vi "generateRTPRBS.vi"(0 "Utilities in":refnum<class "Utilities.lvclass">, 1 "W":dbl=2.0, 3 "Th":dbl=0.02 format="%#_13g", 5 "MAX":dbl=3.0 format="%#_13g", 7 "activate":bool, 9 "MIN":dbl=2.0 format="%#_13g", 11 "error in (no error)":errorcluster, 12 "PRBS samples":i32=800) -> (4 "Utilities out":refnum<class "Utilities.lvclass">, 6 "Val":dbl, 8 "Size":i32, 10 "totalSize":i32, 15 "error out":errorcluster)   [LabVIEW 2023, in "Utilities.lvclass"]
uses:
  Utilities.lvclass
  <vilib>/Analysis/1siggen.llb/Ramp Pattern by Samples.vi
  <vilib>/numeric/Random Number (Range) I64.vi
  <vilib>/numeric/sub_Random U32.vi
  <vilib>/Analysis/1siggen.llb/Ramp Pattern by Delta.vi
  <vilib>/Analysis/NI_AALBase.lvlib
  <vilib>/ptbypt/NI_PtbyPt.lvlib
panel:
  in  "Save":bool
  in  "stop":bool
  out "element":dbl
  out "XY Graph":cluster{dbl, dbl}[](graph)
  out "cos(x)":dbl[](array[numeric])
  in  "time":dbl=0.2 format="%#_13g"
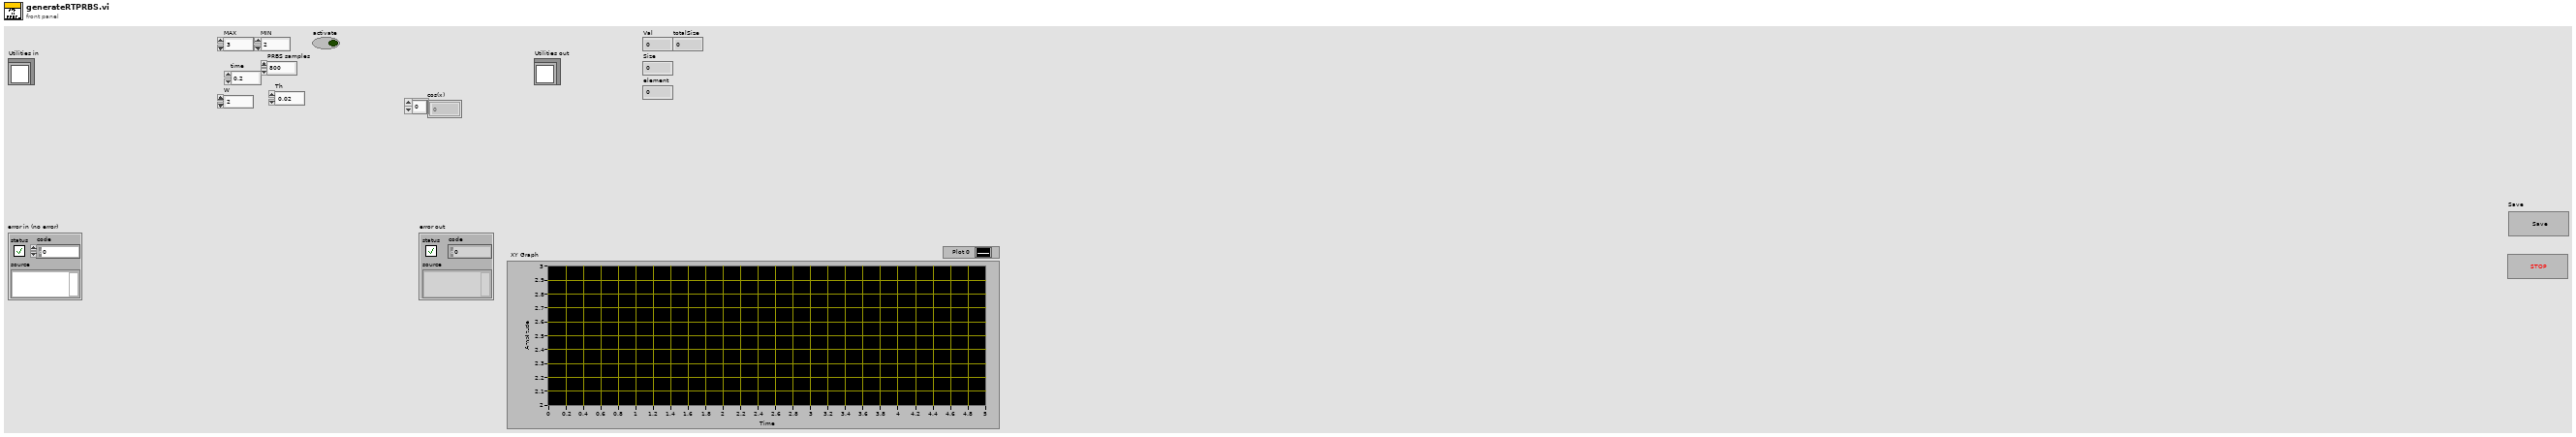
[diagram p1: front panel]
types:
  T1 = typedef "imagedata.ctl" = cluster{"image type":i32, "image depth":i32, "image":u8[], "mask":u8[], "colors":u32[], "Rectangle":cluster{"left":i16, "top":i16, "right":i16, "bottom":i16}}
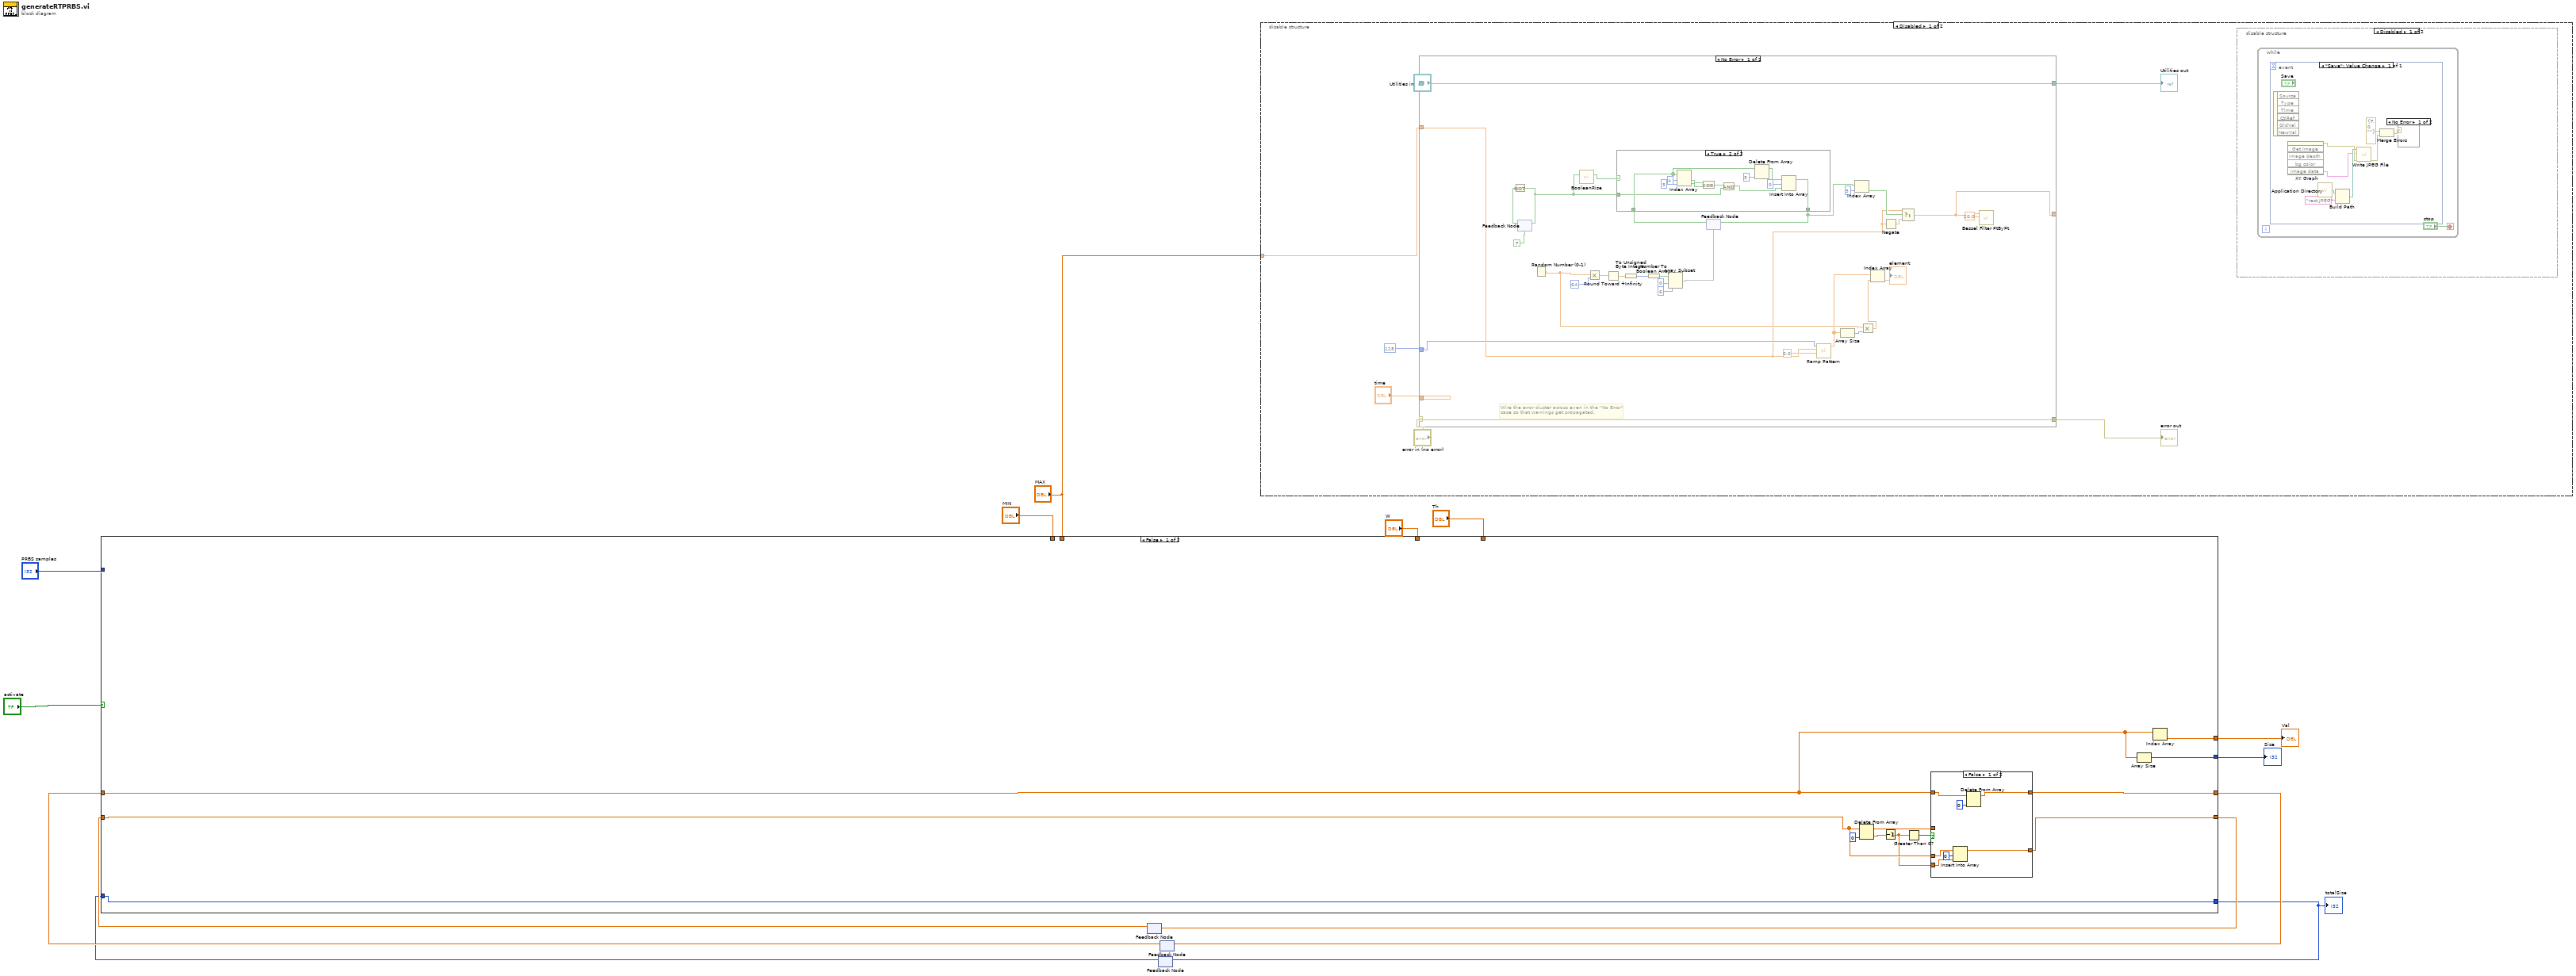
[diagram p0: block diagram]
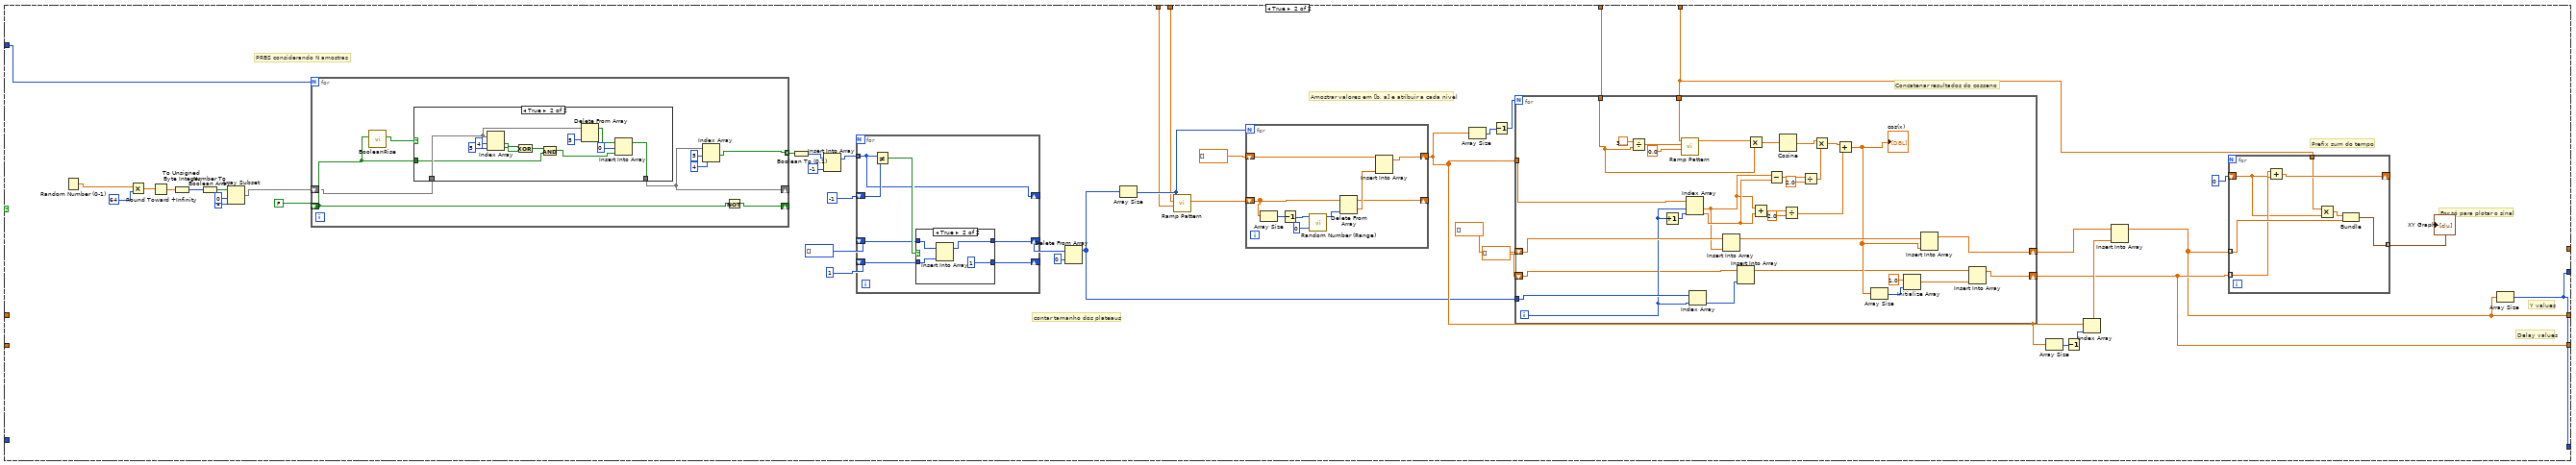
[diagram p8: hidden frame]
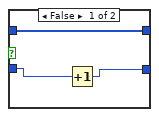
[diagram p10: hidden frame]
diagram:
  n1 = feedback #1() -> (w13:dbl[])  [unwired: 1 in]
  n2 = feedback #2() -> (w1:i32)  [unwired: 1 in]
  n3 = feedback #3() -> (w11:dbl[])  [unwired: 1 in]
  n4 = case shown="False" "activate" {
    tunnel: [w19 w37] -> w12
    tunnel: [w21 w44] -> w14
    tunnel: w13 -> [w23 _]
    tunnel: w11 -> [w17 _]
    tunnel: [w18 _] -> w3
    tunnel: "Th" -> [_ w42]
    tunnel: "W" -> [_ w41]
    tunnel: "MAX" -> [_ w40]
    tunnel: "MIN" -> [_ w39]
    tunnel: "PRBS samples" -> [_ w38]
    tunnel: [w16 w36] -> w5
    tunnel: [w15 w36] -> w2
    tunnel: w1 -> [w15 _]
    frame False {
      n5 = Delete From Array(array=w23, index=0) -> (deleted portion=w26:dbl, array with subset deleted=w24:dbl[])  [unwired: 1 in]
      n6 = Decrement(x=w26) -> (x-1=w22:dbl)
      n7 = Greater Than 0?(x=w22) -> (x > 0?=w25:bool)
      n8 = case shown="False" w25 {
        tunnel: w24 -> [_ w35]
        tunnel: w23 -> [w33 _]
        tunnel: w22 -> [w32 _]
        tunnel: [w31 w35] -> w21
        tunnel: w17 -> [w29 w34]
        tunnel: [w27 w34] -> w19
        frame False {
          n9 = Insert Into Array(array=w33, index=0, new element=w32) -> (w31:dbl[])
          n10 = Delete From Array(array=w29, index=0) -> (array with subset deleted=w27:dbl[])  [unwired: 1 in, 1 out]
        }
        frame True {
        }
      }
      n11 = Array Size(array=w17) -> (size(s)=w16:i32)
      n12 = Index Array(array=w17) -> (element=w18:dbl)  [unwired: 1 in]
    }
    frame True {
      # "For só para plotar o sinal"
      # "Delay values"
      # "Y values"
      # "Prefix sum do tempo"
      # "Concatenar resultados do cosseno"
      # "Amostrar valores em [b, a] e atribuir a cada nivel"
      # "contar tamanho dos plateaus"
      # "PRBS considerando N amostras"
      n13 = Random Number (0-1)() -> (number: 0 to 1=w48:dbl)
      n14 = Multiply(x=w48, y=64) -> (x*y=w71:dbl)
      n15 = Round Toward +Infinity(x=w71) -> (ceil(x): smallest int >= x=w73:dbl)
      n16 = To Unsigned Byte Integer(number=w73) -> (unsigned 8bit integer=w74:u8)
      n17 = Number To Boolean Array(number=w74) -> (Boolean array=w75:bool[])
      n18 = Array Subset(array=w75, index=0, length=6) -> (w49:bool[])
      n19 = for {
        N: w38 -> [_]
        shift-right: [w91] -> _
        shift-left: FALSE -> [w92]
        tunnel: [w89] -> w64 mode=indexing
        shift-right: [w88] -> _
        shift-left: w49 -> [w87]
        n20 = call "BooleanRise.vi"("Boolean in"=w92) -> ("Boolean"=w93:bool)  [unwired: 8 in, 2 out]
        n21 = case shown="True" w93 {
          tunnel: [w95 w106] -> w88
          tunnel: w87 -> [w95 w98]
          tunnel: w92 -> [_ w96]
          frame False {
          }
          frame True {
            n22 = Index Array(array=w98, index #1=4 ("index"), index #2=5 ("index")) -> (element #1=w101:bool, element #2=w102:bool)
            n23 = Exclusive Or(1:w102, 2:w101) -> (0:w97:bool)
            n24 = And(x=w97, y=w96) -> ()  [unwired: 1 out]
            n25 = Delete From Array(array=w98, index=5) -> (array with subset deleted=w104:bool[])  [unwired: 1 in, 1 out]
            n26 = Insert Into Array(array=w104, index=0, new element=w97) -> (w106:bool[])
          }
        }
        n27 = Index Array(array=w88, index #1=5 ("index"), index #2=4 ("index")) -> (element #1=w89:bool)  [unwired: 1 out]
        n28 = Not(x=w92) -> (.not. x?=w91:bool)
      }
      n29 = Boolean To (0,1)(Boolean=w64) -> (0, 1=w63:i16[])
      n30 = Insert Into Array(array=w63, new element=i16 -1 ("new element/subarray")) -> (w61:i16[])  [unwired: 1 in]
      n31 = for {
        shift-right: [w146] -> _
        shift-left: -1 -> [w152]
        shift-right: [w147] -> _
        shift-left: 1 -> [w150]
        shift-right: [w148] -> w66
        shift-left: i32[] [] -> [w149]
        tunnel: w61 -> [w146] mode=indexing
        n32 = Not Equal?(x=w146, y=w152) -> (x != y?=w151:bool)
        n33 = case shown="True" w151 {
          tunnel: w150 -> [w155 w158]
          tunnel: w149 -> [w153 w159]
          tunnel: [w153 w157] -> w148
          tunnel: [w154 1] -> w147
          frame False {
            n34 = Increment(x=w155) -> (x+1=w154:i32)
          }
          frame True {
            n35 = Insert Into Array(array=w159, new element=w158) -> (w157:i32[])  [unwired: 1 in]
          }
        }
      }
      n36 = Delete From Array(array=w66, index=0) -> (array with subset deleted=w46:i32[])  [unwired: 1 in, 1 out]
      n37 = Array Size(array=w46) -> (size(s)=w47:i32)
      n38 = call-poly <vilib>:"Ramp Pattern.vi"("start"=w39, "end"=w40, "samples"=w47) -> ("Ramp Pattern"=w60:dbl[])  [unwired: 7 in, 1 out]
      n39 = for {
        N: w47 -> [_]
        shift-right: [w83] -> _
        shift-left: w60 -> [w80]
        shift-right: [w84] -> w53
        shift-left: dbl[] [] ("Ramp Pattern") -> [w86]
        n40 = Array Size(array=w80) -> (size(s)=w82:i32)
        n41 = Decrement(x=w82) -> (x-1=w81:i32)
        n42 = call-poly <vilib>:"Random Number (Range).vi"("lower bound (-100)"=i64 0, "upper bound (100)"=w81) -> ("number"=w78:i64)  [unwired: 9 in]
        n43 = Delete From Array(array=w80, index=w78) -> (deleted portion=w85:dbl, array with subset deleted=w83:dbl[])  [unwired: 1 in]
        n44 = Insert Into Array(array=w86, new element=w85) -> (w84:dbl[])  [unwired: 1 in]
      }
      n45 = Array Size(array=w53) -> (size(s)=w58:i32)
      n46 = Decrement(x=w58) -> (x-1=w57:i32)
      n47 = for {
        N: w57 -> [_]
        tunnel: w53 -> [w145]
        tunnel: w41 -> [w132]
        tunnel: w42 -> [w129]
        shift-right: [w124] -> w44
        shift-left: dbl[] [] -> [w116]
        shift-right: [w119] -> w55
        shift-left: dbl[] [] ("Ramp Pattern") -> [w123]
        tunnel: w46 -> [w118]
        i -> [w117]
        n48 = Divide(x=3.141592653589793, y=w132) -> (x/y=w135:dbl)
        n49 = Increment(x=w117) -> (x+1=w144:i32)
        n50 = call-poly <vilib>:"Ramp Pattern.vi"("start"=0.0, "end"=w135, "delta"=w129) -> ("Ramp Pattern"=w136:dbl[])  [unwired: 6 in, 2 out]
        n51 = Index Array(array=w145, index #1=w117, index #2=w144) -> (element #1=w122:dbl, element #2=w128:dbl)
        n52 = Index Array(array=w118, index=w117) -> (element=w115:i32)
        n53 = Insert Into Array(array=w123, new element=w122) -> (w121:dbl[])  [unwired: 1 in]
        n54 = Insert Into Array(array=w116, new element=w115) -> (w114:dbl[])  [unwired: 1 in]
        n55 = Multiply(x=w136, y=w132) -> (x*y=w137:dbl[])
        n56 = Add(x=w122, y=w128) -> (x+y=w138:dbl)
        n57 = Subtract(x=w122, y=w128) -> (x-y=w139:dbl)
        n58 = Cosine(x=w137) -> (cos(x)=w140:dbl[])
        n59 = Divide(x=w138, y=2.0) -> (x/y=w143:dbl)
        n60 = Divide(x=w139, y=2.0) -> (x/y=w141:dbl)
        n61 = Multiply(x=w140, y=w141) -> (x*y=w142:dbl[])
        n62 = Add(x=w142, y=w143) -> (x+y=w120:dbl[])
        "cos(x)" <- w120
        n63 = Array Size(array=w120) -> (size(s)=w126:i32)
        n64 = Initialize Array(1.0 ("element"), w126) -> (w125:dbl[])
        n65 = Insert Into Array(array=w121, new element=w120) -> (w119:dbl[])  [unwired: 1 in]
        n66 = Insert Into Array(array=w114, new element=w125) -> (w124:dbl[])  [unwired: 1 in]
      }
      n67 = Array Size(array=w53) -> (size(s)=w52:i32)
      n68 = Decrement(x=w52) -> (x-1=w51:i32)
      n69 = Index Array(array=w53, index=w51) -> (element=w54:dbl)
      n70 = Insert Into Array(array=w55, new element=w54) -> (w37:dbl[])  [unwired: 1 in]
      n71 = for {
        tunnel: w37 -> [w112] mode=indexing
        tunnel: w44 -> [w111] mode=indexing
        tunnel: [w113] -> w43 mode=indexing
        shift-right: [w110] -> _
        shift-left: 0 -> [w109]
        tunnel: w42 -> [w108]
        n72 = Add(x=w109, y=w111) -> (x+y=w110:dbl)
        n73 = Multiply(x=w108, y=w109) -> (x*y=w107:dbl)
        n74 = Bundle(w107, w112) -> (w113:cluster{dbl, dbl})  [unwired: 1 in]
      }
      "XY Graph" <- w43
      n75 = Array Size(array=w37) -> (size(s)=w36:i32)
    }
  }
  "Val" <- w3
  "Size" <- w5
  "totalSize" <- w2
  n76 = feedback-in #1(w14) -> ()
  n77 = feedback-in #2(w2) -> ()
  n78 = feedback-in #3(w12) -> ()
  n79 = disable-structure shown="Disabled" {
    disable-tunnel: "MAX" -> [w160 _]
    frame Disabled {
      n80 = case shown="No Error" "error in (no error)" {
        selector: "error in (no error)" -> [w203 w218]
        tunnel: [w203 w218] -> w165
        tunnel: [w204 w217] -> w163
        tunnel: "Utilities in" -> [w204 w217]
        tunnel: w160 -> [w177 _]
        tunnel: "time" -> [_ _]
        tunnel: 128 -> [w185 _]
        tunnel: [w178 _] -> _
        frame No Error {
          # "Wire the error cluster across even in the \"No Error\"\ncase so that warnings get propagated."
          n81 = feedback #4(FALSE) -> (w191:bool)
          n82 = Not(x=w191) -> (.not. x?=w186:bool)
          n83 = feedback-in #4(w186) -> ()
          n84 = Random Number (0-1)() -> (number: 0 to 1=w181:dbl)
          n85 = call "BooleanRise.vi"("Boolean in"=w186) -> ("Boolean"=w187:bool)  [unwired: 8 in, 2 out]
          n86 = Multiply(x=w181, y=64) -> (x*y=w193:dbl)
          n87 = Round Toward +Infinity(x=w193) -> (ceil(x): smallest int >= x=w195:dbl)
          n88 = To Unsigned Byte Integer(number=w195) -> (unsigned 8bit integer=w196:u8)
          n89 = Number To Boolean Array(number=w196) -> (Boolean array=w197:bool[])
          n90 = Array Subset(array=w197, index=0, length=6) -> (w200:bool[])
          n91 = feedback #5(w200) -> (w201:bool[])
          n92 = case shown="True" w187 {
            tunnel: [w205 w216] -> w190
            tunnel: w201 -> [w205 w208]
            tunnel: w186 -> [_ w206]
            frame False {
            }
            frame True {
              n93 = Index Array(array=w208, index #1=4 ("index"), index #2=5 ("index")) -> (element #1=w211:bool, element #2=w212:bool)
              n94 = Exclusive Or(1:w212, 2:w211) -> (0:w207:bool)
              n95 = And(x=w207, y=w206) -> ()  [unwired: 1 out]
              n96 = Delete From Array(array=w208, index=5) -> (array with subset deleted=w214:bool[])  [unwired: 1 in, 1 out]
              n97 = Insert Into Array(array=w214, index=0, new element=w207) -> (w216:bool[])
            }
          }
          n98 = feedback-in #5(w190) -> ()
          n99 = call-poly <vilib>:"Ramp Pattern.vi"("start"=0.0, "end"=w177, "samples"=w185) -> ("Ramp Pattern"=w183:dbl[])  [unwired: 7 in, 1 out]
          n100 = Array Size(array=w183) -> (size(s)=w182:i32)
          n101 = Index Array(array=w190, index=5) -> (element=w188:bool)
          n102 = Multiply(x=w181, y=w182) -> (x*y=w180:dbl)
          n103 = Index Array(array=w183, index=w180) -> (element=→"element":dbl)
          n104 = Negate(x=w177) -> (-x=w202:dbl)
          n105 = Select(t=w177, s=w188, f=w202) -> (s? t:f=w178:dbl)
          n106 = call <vilib>:"Bessel Filter PtByPt.vi"("sampling freq: fs"=20.0, "x"=w178) -> ()  [unwired: 7 in, 2 out]
        }
        frame Error {
        }
      }
      "error out" <- w165
      "Utilities out" <- w163
      n107 = disable-structure shown="Disabled" {
        frame Disabled {
          n108 = while {
            stop <- "stop" stop-if-true
            n109 = event shown="[0] \"Save\": Value Change" {
              selector: _ -> [_]
              dyn-events: _ -> [_]
              timeout: _ -> [_]
              event "Save": Value Change {
                n110 = event-data() -> ()  [unwired: 1 in, 6 out]
                n111 = invoke on="XY Graph" class="XYGraph (strict)" method="Get Image"() -> (error out=w170:errorcluster, "image data"=w169:T1)  [unwired: 6 in, 4 out]
                n112 = call <vilib>:"Application Directory.vi"() -> ("Application Directory"=w173:path)
                n113 = Build Path(base path=w173, name or relative path="rect.JPEG") -> (appended path=w172:path)
                n114 = call <vilib>:"Write JPEG File.vi"("error in (no error)"=w170, "image data"=w169, "path to JPEG file"=w172) -> ("error out"=w175:errorcluster)  [unwired: 7 in, 1 out]
                n115 = Merge Errors(errorcluster {"status"=FALSE, "code"=0, "source"=""} ("error in"), w175) -> (w171:errorcluster)
                n116 = case shown="No Error" w171 {
                  frame No Error {
                  }
                  frame Error {
                  }
                }
              }
            }
          }
        }
        frame Enabled {
        }
      }
    }
    frame Enabled {
    }
  }
